vi "Begin.vi"(8 "error in":errorcluster) -> (0 "error out":errorcluster)   [LabVIEW 2016]
doc: "Called before other user functions, this VI is expected to open initial I/O refnums, load in file data, and do all program initialization. Notice that the <B>error out</B> terminal is simply used for data flow. Wiring it to other structures or subVIs ensures that this VI runs first."
uses:
  <vilib>/Rock Robotics/WPI/Joystick/WPI_JoystickDeviceEnum.ctl
  <vilib>/Rock Robotics/SystemInterfaces/DIO/FPGA_DIOChannel.ctl
  <vilib>/Rock Robotics/WPI/Solenoid/WPI_SolenoidChannel.ctl
  <vilib>/Rock Robotics/SystemInterfaces/DIO/FPGA_DIOPWMChannel.ctl
  <vilib>/Rock Robotics/WPI/ThirdParty/CanMotor/TalonSRX/WPI_CANTalonSRX_APIControlMode.ctl
  <vilib>/Rock Robotics/WPI/Counter/WPI_CounterDigitalInputToDigitalSource.vi
  <vilib>/Rock Robotics/WPI/Solenoid/WPI_SolenoidOpenSingle.vi
  <vilib>/Rock Robotics/WPI/RobotDrive/WPI_RobotDriveOpen4MotorWithSPARK.vi
  <vilib>/Rock Robotics/WPI/Utilities/WPI_GetSetVariantRefNum.vi
  <vilib>/Rock Robotics/WPI/Switch/WPI_SwitchOpenLimit.vi
  Robot Global Data.vi
  <vilib>/Rock Robotics/WPI/RobotDrive/WPI_RobotDriveOpen2MotorWithSPARK.vi
  <vilib>/Rock Robotics/WPI/MotorControl/WPI_MotorControlOpen SPARK.vi
  <vilib>/Rock Robotics/WPI/RobotDrive/WPI_RobotDriveOpen2MotorWithJaguar.vi
  <vilib>/Rock Robotics/WPI/MotorControl/WPI_MotorControlOpen Jaguar.vi
panel:
  in  "error in 2":errorcluster
  out "error out 2":errorcluster
  # "NOTICE-THIS IS PROTOTYPE CODE!\nIf you want to make revisions to the competition code, please edit the files in the RobotDrive repo"
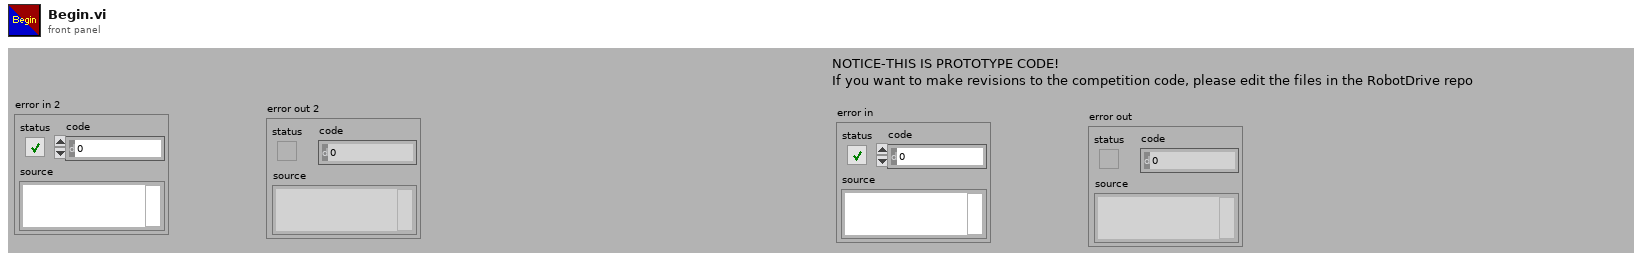
[diagram p1: front panel]
types:
  T1 = typedef "WPI_SolenoidChannel.ctl" = enum8{"Solenoid 0", "Solenoid 1", "Solenoid 2", "Solenoid 3", "Solenoid 4", "Solenoid 5", "Solenoid 6", "Solenoid 7", "Invalid"}
  T2 = typedef "FPGA_DIOChannel.ctl" = enum8{"DIO 0", "DIO 1", "DIO 2", "DIO 3", "DIO 4", "DIO 5", "DIO 6", "DIO 7", "DIO 8", "DIO 9", "DIO MXP 0", "DIO MXP 1", "DIO MXP 2", "DIO MXP 3", "DIO MXP 4", "DIO MXP 5", "DIO MXP 6", "DIO MXP 7", "DIO MXP 8", "DIO MXP 9", "DIO MXP 10", "DIO MXP 11", "DIO MXP 12", "DIO MXP 13", "DIO MXP 14", "DIO MXP 15", "SPI Port CS1", "SPI Port CS2", "SPI Port CS3", "SPI Port MISO", "SPI Port MOSI", "Invalid"}
  T3 = typedef "WPI_CANTalonSRX_APIControlMode.ctl" = enum8{"Percent VBus", "Speed", "Position", "Slave", "Unchanged / Invalid", "Voltage Compensation", "Current", "Motion Profile", "Motion Magic"}
  T4 = typedef "FPGA_DIOPWMChannel.ctl" = enum8{"PWM 0", "PWM 1", "PWM 2", "PWM 3", "PWM 4", "PWM 5", "PWM 6", "PWM 7", "PWM 8", "PWM 9", "PWM MXP 0", "PWM MXP 1", "PWM MXP 2", "PWM MXP 3", "PWM MXP 4", "PWM MXP 5", "PWM MXP 6", "PWM MXP 7", "PWM MXP 8", "PWM MXP 9", "Invalid"}
  T5 = typedef "WPI_JoystickDeviceEnum.ctl" = enum16{"USB 0", "USB 1", "USB 2", "USB 3", "USB 4", "USB 5"}
  T6 = typedef "WPI_JoystickDevRef.ctl" = cluster{"Device":T5}
  T7 = typedef "WPI_RobotDriveDevRef.ctl" = cluster{"DevStatus":errorcluster, "Motors[]":T8[], "Square Inputs":bool, "Max Output":dbl}
  T8 = typedef "WPI_MotorControlDeviceRef.ctl" = cluster{"DeviceStatus":errorcluster, "Type":T9, "PWM":cluster{"PWM Channel":T4, "DeadBand":T10}, "CAN":cluster{"Device Number":u8, "SetOutput VI Ref":variant, "GetOutput VI Ref":variant, "Enable VI Ref":variant, "Disable VI Ref":variant, "Data":variant}, "Invert":bool}
  T9 = typedef "WPI_MotorControlType.ctl" = enum16{"PWM", "CAN"}
  T10 = typedef "WPI_PWMDeadband.ctl" = cluster{"Name":string, "maxPositivePwm":i32, "minPositivePwm":i32, "centerPwm":i32, "maxNegativePwm":i32, "minNegativePwm":i32, "angularRange":u16}
  T11 = typedef "WPI_DigitalInputDevRef.ctl" = cluster{"DevStatus":errorcluster, "DIO Channel":T2}
  T12 = typedef "FPGA_CounterEncoderSourceConvertionLVSourceType.ctl" = cluster{"DevStatus":errorcluster, "AnalogTriggerMode?":bool, "DigitalMode":cluster{"DIO Channel":T13}, "AnalogTriggerMode":cluster{"AnalogTriggerIndex":T14, "OutputType":T15}}
  T13 = typedef "FPGA_DIODigitalSourceChannel.ctl" = enum8{"DIO 0", "DIO 1", "DIO 2", "DIO 3", "DIO 4", "DIO 5", "DIO 6", "DIO 7", "DIO 8", "DIO 9", "DIO MXP 0", "DIO MXP 1", "DIO MXP 2", "DIO MXP 3", "DIO MXP 4", "DIO MXP 5", "DIO MXP 6", "DIO MXP 7", "DIO MXP 8", "DIO MXP 9", "DIO MXP 10", "DIO MXP 11", "DIO MXP 12", "DIO MXP 13", "DIO MXP 14", "DIO MXP 15", "Disabled"}
  T14 = typedef "FPGA_AnalogTriggerIndex.ctl" = enum8{"Trig 0", "Trig 1", "Trig 2", "Trig 3", "Trig 4", "Trig 5", "Trig 6", "Trig 7", "Invalid"}
  T15 = typedef "FPGA_AnalogTriggerOutType.ctl" = enum16{"InWindow", "TriggerState", "Rising", "Falling"}
  T16 = typedef "WPI_EncoderDevRef.ctl" = cluster{"DevStatus":errorcluster, "EncoderIndex":T17, "CounterIndex":T18, "DistancePerCount":dbl, "Decoding Type":T19}
  T17 = typedef "FPGA_EncoderIdx.ctl" = enum8{"Enc 0", "Enc 1", "Enc 2", "Enc 3", "Enc 4", "Enc 5", "Enc 6", "Enc 7", "Invalid"}
  T18 = typedef "FPGA_CounterCtrSystemIndex.ctl" = enum8{"Ctr 0", "Ctr 1", "Ctr 2", "Ctr 3", "Ctr 4", "Ctr 5", "Ctr 6", "Ctr 7", "Invalid"}
  T19 = typedef "WPI_EncoderType.ctl" = enum16{"1x", "2x", "4x"}
  T20 = typedef "WPI_SolenoidDevRef.ctl" = cluster{"DevStatus":errorcluster, "Pneumatics Control Module":u8, "Forward Solenoid Channel":T1, "Reverse Solenoid Channel":T1}
  T21 = typedef "WPI_CompressorDevRef.ctl" = cluster{"DevStatus":errorcluster, "Pneumatics Control Module":u8}
  T22 = typedef "WPI_CameraDevRef.ctl" = cluster{"Camera Address":string, "CameraStatus":errorcluster}
  T23 = typedef "WPI_SwitchDevRef.ctl" = cluster{"DevStatus":errorcluster, "DIO Channel":T2, "CntIndex":T18, "Normally Closed":bool}
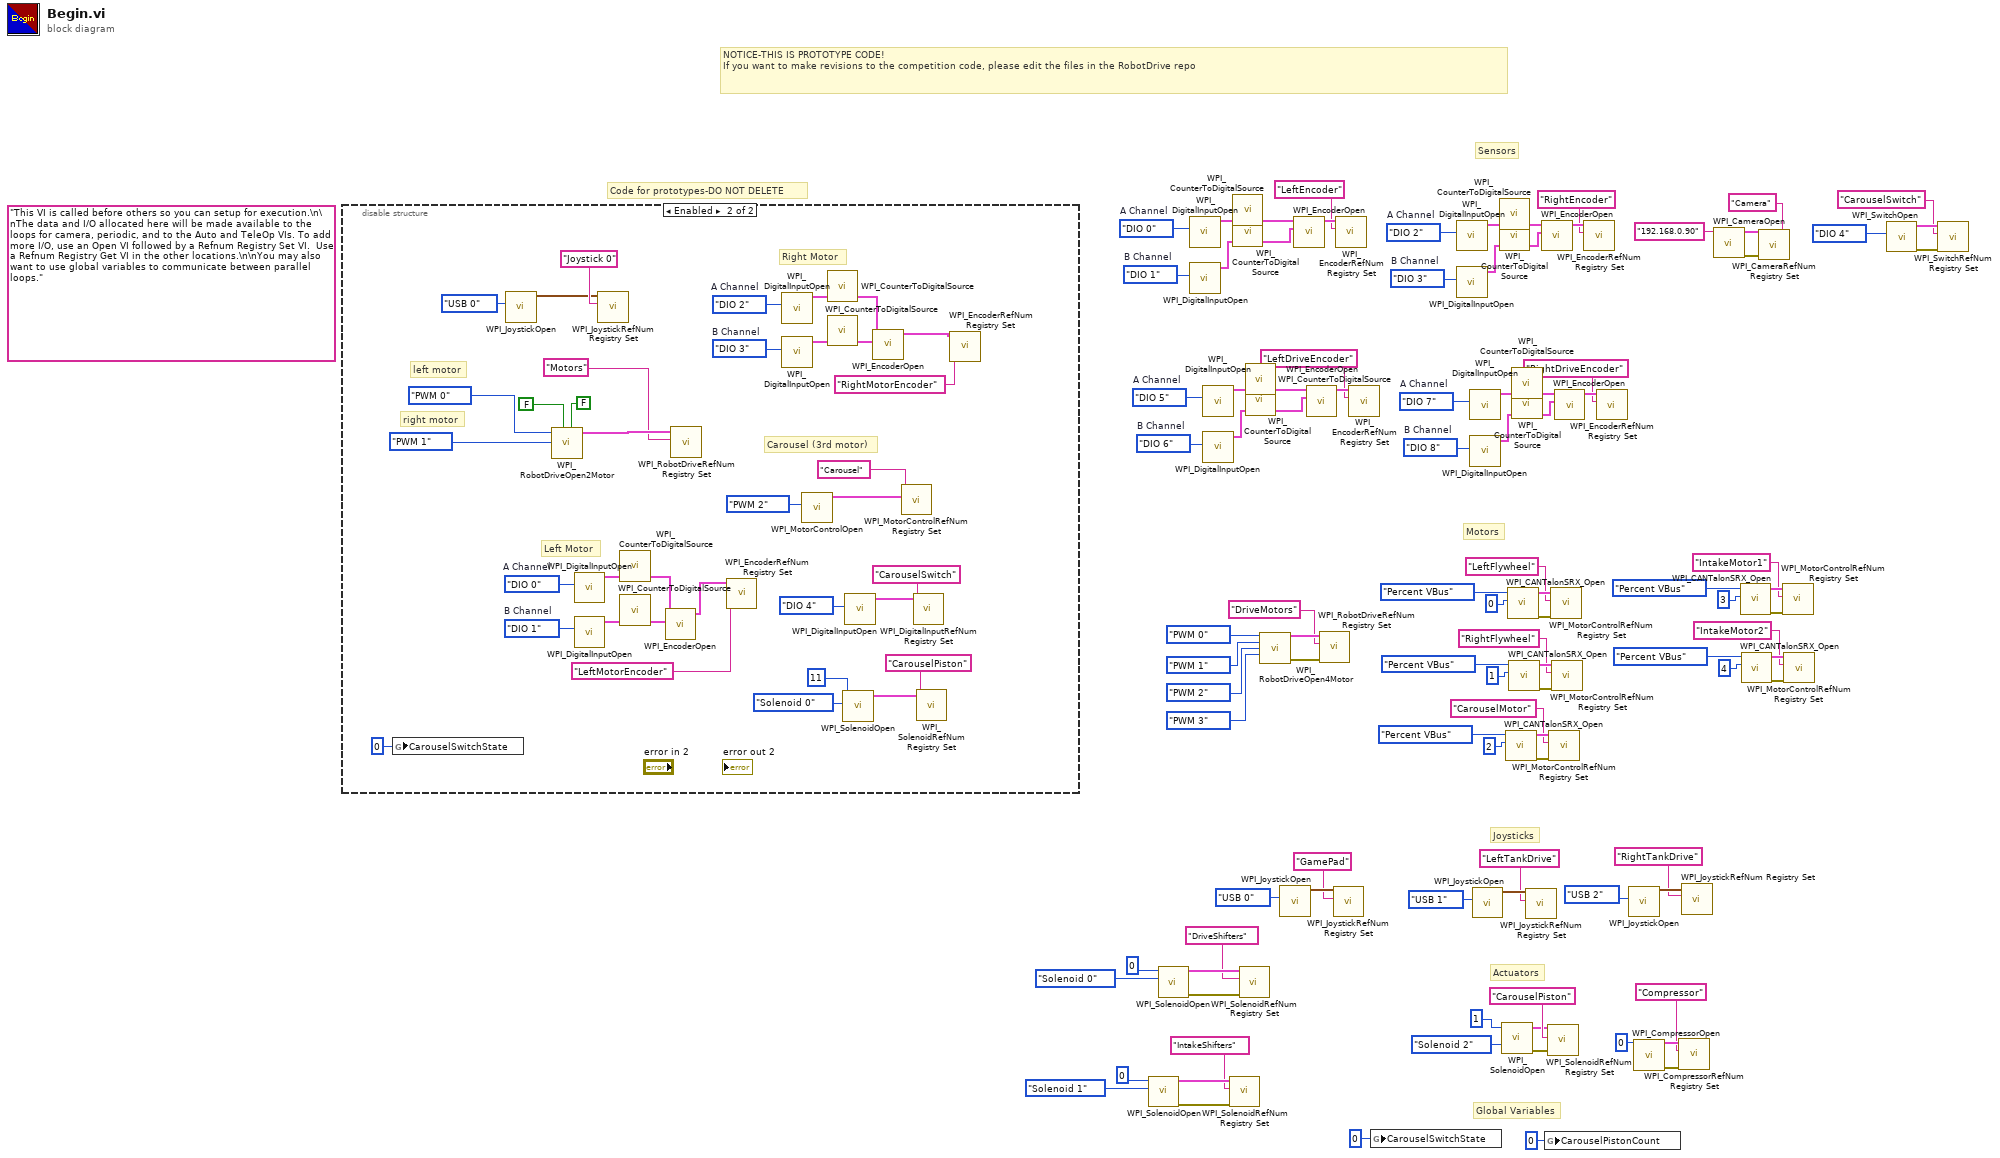
[diagram p0: block diagram]
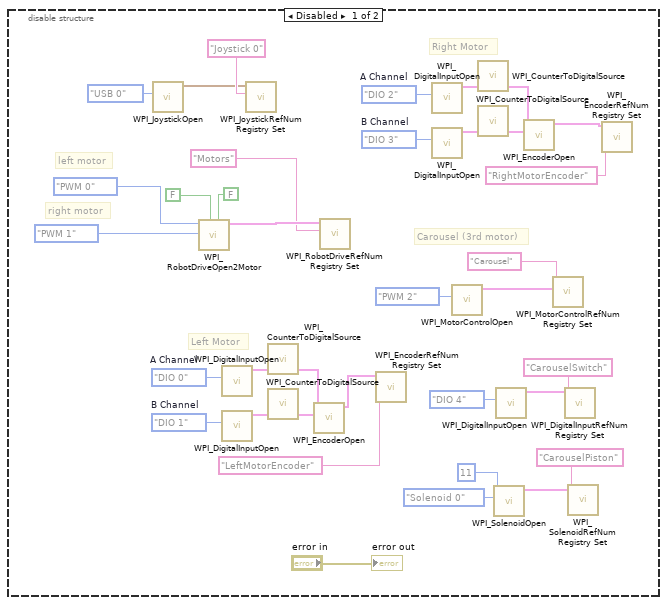
[diagram p2: hidden frame]
diagram:
  w13 = FPGA_DIOChannel."DIO 8"  # B Channel
  w12 = FPGA_DIOChannel."DIO 7"  # A Channel
  w21 = FPGA_DIOChannel."DIO 6"  # B Channel
  w20 = FPGA_DIOChannel."DIO 5"  # A Channel
  w81 = FPGA_DIOChannel."DIO 3"  # B Channel
  w80 = FPGA_DIOChannel."DIO 2"  # A Channel
  w89 = FPGA_DIOChannel."DIO 1"  # B Channel
  w88 = FPGA_DIOChannel."DIO 0"  # A Channel
  (unwired) "This VI is called before others so you can setup for execution.\n\nThe data and I/O allocated here will be made available to the loops for camera, periodic, and to the Auto and TeleOp VIs. To add more I/O, use an Open VI followed by a Refnum Registry Set VI.  Use a Refnum Registry Get VI in the other locations.\n\nYou may also want to use global variables to communicate between parallel loops."
  # "Global Variables"
  # "Actuators"
  # "Joysticks"
  # "Motors"
  # "Sensors"
  # "NOTICE-THIS IS PROTOTYPE CODE!\nIf you want to make revisions to the competition code, please edit the files in the RobotDrive repo"
  # "Code for prototypes-DO NOT DELETE"
  n1 = disable-structure shown="Enabled" {
    frame Disabled {
      w124 = FPGA_DIOChannel."DIO 3"  # B Channel
      w123 = FPGA_DIOChannel."DIO 2"  # A Channel
      w132 = FPGA_DIOChannel."DIO 1"  # B Channel
      w131 = FPGA_DIOChannel."DIO 0"  # A Channel
      # "Carousel (3rd motor)"
      # "Right Motor"
      # "right motor"
      # "left motor"
      # "Left Motor"
      n2 = call <vilib>:"WPI_JoystickOpen.vi"("JoystickDevice"=WPI_JoystickDeviceEnum."USB 0") -> ("JoystickDevRef"=w110:T6)  [unwired: 10 in]
      n3 = call-poly <vilib>:"WPI_RobotDriveOpen2Motor.vi"("Right Motor Inverted"=FALSE, "Left Motor Inverted"=FALSE, "Right Motor"=FPGA_DIOPWMChannel."PWM 1", "Left Motor"=FPGA_DIOPWMChannel."PWM 0") -> ("RobotDriveDevRef"=w134:T7)  [unwired: 6 in, 1 out]
      n4 = call <vilib>:"WPI_DigitalInputOpen.vi"("DIO Channel"=w131) -> ("DigitalInputDevRef"=w128:T11)  [unwired: 1 in, 9 out]
      n5 = call <vilib>:"WPI_DigitalInputOpen.vi"("DIO Channel"=w132) -> ("DigitalInputDevRef"=w129:T11)  [unwired: 1 in, 9 out]
      n6 = call <vilib>:"WPI_JoystickRefNum Registry Set.vi"("refnum name"="Joystick 0", "JoystickDevRef"=w110) -> ()  [unwired: 8 in, 2 out]
      n7 = call-poly <vilib>:"WPI_CounterToDigitalSource.vi"("DigitalInputDevRef"=w128) -> ("Digital Source"=w127:T12)  [unwired: 6 out]
      n8 = call-poly <vilib>:"WPI_CounterToDigitalSource.vi"("DigitalInputDevRef"=w129) -> ("Digital Source"=w130:T12)  [unwired: 6 out]
      n9 = call <vilib>:"WPI_EncoderOpen.vi"("BSource"=w130, "ASource"=w127) -> ("EncoderDevRef"=w126:T16)  [unwired: 6 in, 3 out]
      n10 = call <vilib>:"WPI_RobotDriveRefNum Registry Set.vi"("refnum name"="Motors", "RobotDriveDevRef"=w134) -> ()  [unwired: 8 in, 2 out]
      n11 = call <vilib>:"WPI_EncoderRefNum Registry Set.vi"("refnum name"="LeftMotorEncoder", "EncoderDevRef"=w126) -> ()  [unwired: 8 in, 2 out]
      n12 = call <vilib>:"WPI_DigitalInputOpen.vi"("DIO Channel"=w123) -> ("DigitalInputDevRef"=w120:T11)  [unwired: 1 in, 9 out]
      n13 = call <vilib>:"WPI_DigitalInputOpen.vi"("DIO Channel"=w124) -> ("DigitalInputDevRef"=w121:T11)  [unwired: 1 in, 9 out]
      n14 = call-poly <vilib>:"WPI_MotorControlOpen.vi"("PWM Channel"=FPGA_DIOPWMChannel."PWM 2") -> ("MotorControlDeviceRef"=w114:T8)  [unwired: 9 in, 1 out]
      n15 = call-poly <vilib>:"WPI_CounterToDigitalSource.vi"("DigitalInputDevRef"=w120) -> ("Digital Source"=w119:T12)  [unwired: 6 out]
      n16 = call-poly <vilib>:"WPI_CounterToDigitalSource.vi"("DigitalInputDevRef"=w121) -> ("Digital Source"=w122:T12)  [unwired: 6 out]
      n17 = call-poly <vilib>:"WPI_SolenoidOpen.vi"("Solenoid Channel"=WPI_SolenoidChannel."Solenoid 0", "Pneumatics Control Module (0)"=u8 11) -> ("SolenoidDevRef"=w106:T20)  [unwired: 8 in, 1 out]
      n18 = call <vilib>:"WPI_DigitalInputOpen.vi"("DIO Channel"=FPGA_DIOChannel."DIO 4") -> ("DigitalInputDevRef"=w108:T11)  [unwired: 9 in, 1 out]
      n19 = call <vilib>:"WPI_EncoderOpen.vi"("BSource"=w122, "ASource"=w119) -> ("EncoderDevRef"=w118:T16)  [unwired: 6 in, 3 out]
      n20 = call <vilib>:"WPI_MotorControlRefNum Registry Set.vi"("refnum name"="Carousel", "MotorControlDevRef"=w114) -> ()  [unwired: 8 in, 2 out]
      n21 = call <vilib>:"WPI_DigitalInputRefNum Registry Set.vi"("refnum name"="CarouselSwitch", "DigitalInputDevRef"=w108) -> ()  [unwired: 8 in, 2 out]
      n22 = call <vilib>:"WPI_SolenoidRefNum Registry Set.vi"("refnum name"="CarouselPiston", "SolenoidDevRef"=w106) -> ()  [unwired: 8 in, 2 out]
      n23 = call <vilib>:"WPI_EncoderRefNum Registry Set.vi"("refnum name"="RightMotorEncoder", "EncoderDevRef"=w118) -> ()  [unwired: 8 in, 2 out]
      "error out" <- "error in"
    }
    frame Enabled {
      w160 = FPGA_DIOChannel."DIO 3"  # B Channel
      w159 = FPGA_DIOChannel."DIO 2"  # A Channel
      w168 = FPGA_DIOChannel."DIO 1"  # B Channel
      w167 = FPGA_DIOChannel."DIO 0"  # A Channel
      # "Carousel (3rd motor)"
      # "Right Motor"
      # "right motor"
      # "left motor"
      # "Left Motor"
      n24 = global write "Robot Global Data.vi" "CarouselSwitchState"(u8 0 ("CarouselSwitchState")) -> ()
      n25 = call <vilib>:"WPI_JoystickOpen.vi"("JoystickDevice"=WPI_JoystickDeviceEnum."USB 0") -> ("JoystickDevRef"=w147:T6)  [unwired: 10 in]
      n26 = call-poly <vilib>:"WPI_RobotDriveOpen2Motor.vi"("Right Motor Inverted"=FALSE, "Left Motor Inverted"=FALSE, "Right Motor"=FPGA_DIOPWMChannel."PWM 1", "Left Motor"=FPGA_DIOPWMChannel."PWM 0") -> ("RobotDriveDevRef"=w170:T7)  [unwired: 6 in, 1 out]
      n27 = call <vilib>:"WPI_DigitalInputOpen.vi"("DIO Channel"=w167) -> ("DigitalInputDevRef"=w164:T11)  [unwired: 1 in, 9 out]
      n28 = call <vilib>:"WPI_DigitalInputOpen.vi"("DIO Channel"=w168) -> ("DigitalInputDevRef"=w165:T11)  [unwired: 1 in, 9 out]
      n29 = call <vilib>:"WPI_JoystickRefNum Registry Set.vi"("refnum name"="Joystick 0", "JoystickDevRef"=w147) -> ()  [unwired: 8 in, 2 out]
      n30 = call-poly <vilib>:"WPI_CounterToDigitalSource.vi"("DigitalInputDevRef"=w164) -> ("Digital Source"=w163:T12)  [unwired: 6 out]
      n31 = call-poly <vilib>:"WPI_CounterToDigitalSource.vi"("DigitalInputDevRef"=w165) -> ("Digital Source"=w166:T12)  [unwired: 6 out]
      n32 = call <vilib>:"WPI_EncoderOpen.vi"("BSource"=w166, "ASource"=w163) -> ("EncoderDevRef"=w162:T16)  [unwired: 6 in, 3 out]
      n33 = call <vilib>:"WPI_RobotDriveRefNum Registry Set.vi"("refnum name"="Motors", "RobotDriveDevRef"=w170) -> ()  [unwired: 8 in, 2 out]
      n34 = call <vilib>:"WPI_EncoderRefNum Registry Set.vi"("refnum name"="LeftMotorEncoder", "EncoderDevRef"=w162) -> ()  [unwired: 8 in, 2 out]
      n35 = call <vilib>:"WPI_DigitalInputOpen.vi"("DIO Channel"=w159) -> ("DigitalInputDevRef"=w156:T11)  [unwired: 1 in, 9 out]
      n36 = call <vilib>:"WPI_DigitalInputOpen.vi"("DIO Channel"=w160) -> ("DigitalInputDevRef"=w157:T11)  [unwired: 1 in, 9 out]
      n37 = call-poly <vilib>:"WPI_MotorControlOpen.vi"("PWM Channel"=FPGA_DIOPWMChannel."PWM 2") -> ("MotorControlDeviceRef"=w151:T8)  [unwired: 9 in, 1 out]
      n38 = call-poly <vilib>:"WPI_CounterToDigitalSource.vi"("DigitalInputDevRef"=w156) -> ("Digital Source"=w155:T12)  [unwired: 6 out]
      n39 = call-poly <vilib>:"WPI_CounterToDigitalSource.vi"("DigitalInputDevRef"=w157) -> ("Digital Source"=w158:T12)  [unwired: 6 out]
      n40 = call-poly <vilib>:"WPI_SolenoidOpen.vi"("Solenoid Channel"=WPI_SolenoidChannel."Solenoid 0", "Pneumatics Control Module (0)"=u8 11) -> ("SolenoidDevRef"=w143:T20)  [unwired: 8 in, 1 out]
      n41 = call <vilib>:"WPI_DigitalInputOpen.vi"("DIO Channel"=FPGA_DIOChannel."DIO 4") -> ("DigitalInputDevRef"=w145:T11)  [unwired: 9 in, 1 out]
      n42 = call <vilib>:"WPI_EncoderOpen.vi"("BSource"=w158, "ASource"=w155) -> ("EncoderDevRef"=w154:T16)  [unwired: 6 in, 3 out]
      n43 = call <vilib>:"WPI_MotorControlRefNum Registry Set.vi"("refnum name"="Carousel", "MotorControlDevRef"=w151) -> ()  [unwired: 8 in, 2 out]
      n44 = call <vilib>:"WPI_DigitalInputRefNum Registry Set.vi"("refnum name"="CarouselSwitch", "DigitalInputDevRef"=w145) -> ()  [unwired: 8 in, 2 out]
      n45 = call <vilib>:"WPI_SolenoidRefNum Registry Set.vi"("refnum name"="CarouselPiston", "SolenoidDevRef"=w143) -> ()  [unwired: 8 in, 2 out]
      n46 = call <vilib>:"WPI_EncoderRefNum Registry Set.vi"("refnum name"="RightMotorEncoder", "EncoderDevRef"=w154) -> ()  [unwired: 8 in, 2 out]
    }
  }
  n47 = call-poly <vilib>:"WPI_SolenoidOpen.vi"("Solenoid Channel"=WPI_SolenoidChannel."Solenoid 1", "Pneumatics Control Module (0)"=u8 0) -> ("error out"=w5:errorcluster, "SolenoidDevRef"=w4:T20)  [unwired: 8 in]
  n48 = call-poly <vilib>:"WPI_SolenoidOpen.vi"("Solenoid Channel"=WPI_SolenoidChannel."Solenoid 0", "Pneumatics Control Module (0)"=u8 0) -> ("error out"=w73:errorcluster, "SolenoidDevRef"=w72:T20)  [unwired: 8 in]
  n49 = call <vilib>:"WPI_DigitalInputOpen.vi"("DIO Channel"=w88) -> ("DigitalInputDevRef"=w85:T11)  [unwired: 1 in, 9 out]
  n50 = call <vilib>:"WPI_DigitalInputOpen.vi"("DIO Channel"=w89) -> ("DigitalInputDevRef"=w86:T11)  [unwired: 1 in, 9 out]
  n51 = call <vilib>:"WPI_DigitalInputOpen.vi"("DIO Channel"=w20) -> ("DigitalInputDevRef"=w17:T11)  [unwired: 1 in, 9 out]
  n52 = call <vilib>:"WPI_DigitalInputOpen.vi"("DIO Channel"=w21) -> ("DigitalInputDevRef"=w18:T11)  [unwired: 1 in, 9 out]
  n53 = call <vilib>:"WPI_SolenoidRefNum Registry Set.vi"("error in (no error)"=w5, "refnum name"="IntakeShifters", "SolenoidDevRef"=w4) -> ()  [unwired: 7 in, 2 out]
  n54 = call-poly <vilib>:"WPI_CounterToDigitalSource.vi"("DigitalInputDevRef"=w85) -> ("Digital Source"=w84:T12)  [unwired: 6 out]
  n55 = call-poly <vilib>:"WPI_CounterToDigitalSource.vi"("DigitalInputDevRef"=w86) -> ("Digital Source"=w87:T12)  [unwired: 6 out]
  n56 = call <vilib>:"WPI_SolenoidRefNum Registry Set.vi"("error in (no error)"=w73, "refnum name"="DriveShifters", "SolenoidDevRef"=w72) -> ()  [unwired: 7 in, 2 out]
  n57 = call-poly <vilib>:"WPI_CounterToDigitalSource.vi"("DigitalInputDevRef"=w17) -> ("Digital Source"=w16:T12)  [unwired: 6 out]
  n58 = call-poly <vilib>:"WPI_CounterToDigitalSource.vi"("DigitalInputDevRef"=w18) -> ("Digital Source"=w19:T12)  [unwired: 6 out]
  n59 = call-poly <vilib>:"WPI_RobotDriveOpen4Motor.vi"("Rear Left Motor"=FPGA_DIOPWMChannel."PWM 0", "Rear Right Motor"=FPGA_DIOPWMChannel."PWM 1", "Front Left Motor"=FPGA_DIOPWMChannel."PWM 2", "Front Right Motor"=FPGA_DIOPWMChannel."PWM 3") -> ("RobotDriveDevRef"=w65:T7, "error out"=w66:errorcluster)  [unwired: 10 in]
  n60 = call <vilib>:"WPI_JoystickOpen.vi"("JoystickDevice"=WPI_JoystickDeviceEnum."USB 0") -> ("JoystickDevRef"=w102:T6)  [unwired: 10 in]
  n61 = call <vilib>:"WPI_EncoderOpen.vi"("BSource"=w87, "ASource"=w84) -> ("EncoderDevRef"=w83:T16)  [unwired: 6 in, 3 out]
  n62 = call <vilib>:"WPI_EncoderOpen.vi"("BSource"=w19, "ASource"=w16) -> ("EncoderDevRef"=w15:T16)  [unwired: 6 in, 3 out]
  n63 = call <vilib>:"WPI_RobotDriveRefNum Registry Set.vi"("error in (no error)"=w66, "refnum name"="DriveMotors", "RobotDriveDevRef"=w65) -> ()  [unwired: 7 in, 2 out]
  n64 = call <vilib>:"WPI_JoystickRefNum Registry Set.vi"("refnum name"="GamePad", "JoystickDevRef"=w102) -> ()  [unwired: 8 in, 2 out]
  n65 = call <vilib>:"WPI_EncoderRefNum Registry Set.vi"("refnum name"="LeftEncoder", "EncoderDevRef"=w83) -> ()  [unwired: 8 in, 2 out]
  n66 = call <vilib>:"WPI_EncoderRefNum Registry Set.vi"("refnum name"="LeftDriveEncoder", "EncoderDevRef"=w15) -> ()  [unwired: 8 in, 2 out]
  n67 = global write "Robot Global Data.vi" "CarouselSwitchState"(u8 0 ("CarouselSwitchState")) -> ()
  n68 = call <vilib>:"WPI_DigitalInputOpen.vi"("DIO Channel"=w80) -> ("DigitalInputDevRef"=w77:T11)  [unwired: 1 in, 9 out]
  n69 = call <vilib>:"WPI_DigitalInputOpen.vi"("DIO Channel"=w81) -> ("DigitalInputDevRef"=w78:T11)  [unwired: 1 in, 9 out]
  n70 = call <vilib>:"WPI_DigitalInputOpen.vi"("DIO Channel"=w12) -> ("DigitalInputDevRef"=w9:T11)  [unwired: 1 in, 9 out]
  n71 = call <vilib>:"WPI_DigitalInputOpen.vi"("DIO Channel"=w13) -> ("DigitalInputDevRef"=w10:T11)  [unwired: 1 in, 9 out]
  n72 = call <vilib>:"WPI_JoystickOpen.vi"("JoystickDevice"=WPI_JoystickDeviceEnum."USB 1") -> ("JoystickDevRef"=w99:T6)  [unwired: 10 in]
  n73 = call-poly <vilib>:"WPI_CounterToDigitalSource.vi"("DigitalInputDevRef"=w77) -> ("Digital Source"=w76:T12)  [unwired: 6 out]
  n74 = call-poly <vilib>:"WPI_CounterToDigitalSource.vi"("DigitalInputDevRef"=w78) -> ("Digital Source"=w79:T12)  [unwired: 6 out]
  n75 = call-poly <vilib>:"WPI_SolenoidOpen.vi"("Solenoid Channel"=WPI_SolenoidChannel."Solenoid 2", "Pneumatics Control Module (0)"=u8 1) -> ("error out"=w27:errorcluster, "SolenoidDevRef"=w26:T20)  [unwired: 8 in]
  n76 = call <vilib>:"WPI_CANTalonSRX_Open.vi"("Device Number"=u8 2, "Control Mode"=WPI_CANTalonSRX_APIControlMode."Percent VBus") -> ("error out"=w45:errorcluster, "CAN Talon SRX Ref"=w44:T8)  [unwired: 8 in]
  n77 = call <vilib>:"WPI_CANTalonSRX_Open.vi"("Device Number"=u8 0, "Control Mode"=WPI_CANTalonSRX_APIControlMode."Percent VBus") -> ("error out"=w55:errorcluster, "CAN Talon SRX Ref"=w54:T8)  [unwired: 8 in]
  n78 = call <vilib>:"WPI_CANTalonSRX_Open.vi"("Device Number"=u8 1, "Control Mode"=WPI_CANTalonSRX_APIControlMode."Percent VBus") -> ("error out"=w50:errorcluster, "CAN Talon SRX Ref"=w49:T8)  [unwired: 8 in]
  n79 = call-poly <vilib>:"WPI_CounterToDigitalSource.vi"("DigitalInputDevRef"=w9) -> ("Digital Source"=w8:T12)  [unwired: 6 out]
  n80 = call-poly <vilib>:"WPI_CounterToDigitalSource.vi"("DigitalInputDevRef"=w10) -> ("Digital Source"=w11:T12)  [unwired: 6 out]
  n81 = call <vilib>:"WPI_JoystickRefNum Registry Set.vi"("refnum name"="LeftTankDrive", "JoystickDevRef"=w99) -> ()  [unwired: 8 in, 2 out]
  n82 = call <vilib>:"WPI_EncoderOpen.vi"("BSource"=w79, "ASource"=w76) -> ("EncoderDevRef"=w75:T16)  [unwired: 6 in, 3 out]
  n83 = global write "Robot Global Data.vi" "CarouselPistonCount"(u8 0 ("CarouselSwitchState")) -> ()
  n84 = call <vilib>:"WPI_SolenoidRefNum Registry Set.vi"("error in (no error)"=w27, "refnum name"="CarouselPiston", "SolenoidDevRef"=w26) -> ()  [unwired: 7 in, 2 out]
  n85 = call <vilib>:"WPI_MotorControlRefNum Registry Set.vi"("error in (no error)"=w45, "refnum name"="CarouselMotor", "MotorControlDevRef"=w44) -> ()  [unwired: 7 in, 2 out]
  n86 = call <vilib>:"WPI_MotorControlRefNum Registry Set.vi"("error in (no error)"=w55, "refnum name"="LeftFlywheel", "MotorControlDevRef"=w54) -> ()  [unwired: 7 in, 2 out]
  n87 = call <vilib>:"WPI_MotorControlRefNum Registry Set.vi"("error in (no error)"=w50, "refnum name"="RightFlywheel", "MotorControlDevRef"=w49) -> ()  [unwired: 7 in, 2 out]
  n88 = call <vilib>:"WPI_EncoderOpen.vi"("BSource"=w11, "ASource"=w8) -> ("EncoderDevRef"=w7:T16)  [unwired: 6 in, 3 out]
  n89 = call <vilib>:"WPI_EncoderRefNum Registry Set.vi"("refnum name"="RightEncoder", "EncoderDevRef"=w75) -> ()  [unwired: 8 in, 2 out]
  n90 = call <vilib>:"WPI_EncoderRefNum Registry Set.vi"("refnum name"="RightDriveEncoder", "EncoderDevRef"=w7) -> ()  [unwired: 8 in, 2 out]
  n91 = call <vilib>:"WPI_JoystickOpen.vi"("JoystickDevice"=WPI_JoystickDeviceEnum."USB 2") -> ("JoystickDevRef"=w96:T6)  [unwired: 10 in]
  n92 = call <vilib>:"WPI_CompressorOpen.vi"("Pneumatics Control Module (0)"=u8 0) -> ("CompressorDevRef"=w67:T21, "error out"=w68:errorcluster)  [unwired: 13 in]
  n93 = call <vilib>:"WPI_CompressorRefNum Registry Set.vi"("error in (no error)"=w68, "refnum name"="Compressor", "CompressorDevRef"=w67) -> ()  [unwired: 7 in, 2 out]
  n94 = call <vilib>:"WPI_JoystickRefNum Registry Set.vi"("refnum name"="RightTankDrive", "JoystickDevRef"=w96) -> ()  [unwired: 8 in, 2 out]
  n95 = call <vilib>:"WPI_CameraOpen.vi"("Camera Address"="192.168.0.90") -> ("error out"=w93:errorcluster, "CameraDevRef"=w92:T22)  [unwired: 9 in]
  n96 = call <vilib>:"WPI_CANTalonSRX_Open.vi"("Device Number"=u8 3, "Control Mode"=WPI_CANTalonSRX_APIControlMode."Percent VBus") -> ("error out"=w40:errorcluster, "CAN Talon SRX Ref"=w39:T8)  [unwired: 8 in]
  n97 = call <vilib>:"WPI_CANTalonSRX_Open.vi"("Device Number"=u8 4, "Control Mode"=WPI_CANTalonSRX_APIControlMode."Percent VBus") -> ("error out"=w35:errorcluster, "CAN Talon SRX Ref"=w34:T8)  [unwired: 8 in]
  n98 = call <vilib>:"WPI_CameraRefNum Registry Set.vi"("error in (no error)"=w93, "refnum name"="Camera", "CameraDevRef"=w92) -> ()  [unwired: 7 in, 2 out]
  n99 = call <vilib>:"WPI_MotorControlRefNum Registry Set.vi"("error in (no error)"=w40, "refnum name"="IntakeMotor1", "MotorControlDevRef"=w39) -> ()  [unwired: 7 in, 2 out]
  n100 = call <vilib>:"WPI_MotorControlRefNum Registry Set.vi"("error in (no error)"=w35, "refnum name"="IntakeMotor2", "MotorControlDevRef"=w34) -> ()  [unwired: 7 in, 2 out]
  n101 = call-poly <vilib>:"WPI_SwitchOpen.vi"("DIO Channel"=FPGA_DIOChannel."DIO 4") -> ("error out"=w32:errorcluster, "SwitchDevRef"=w31:T23)  [unwired: 9 in]
  n102 = call <vilib>:"WPI_SwitchRefNum Registry Set.vi"("error in (no error)"=w32, "refnum name"="CarouselSwitch", "SwitchDevRef"=w31) -> ()  [unwired: 7 in, 2 out]
